vi "Simple TCP - Server.vi"() -> ()   [LabVIEW 2020]
doc: "Demonstrates how to set up a basic TCP connection, send data to the specified port once a connection has been established, and terminate the connection once the data has been sent. This VI is designed to stop if the TCP connection is terminated. The data sent in this example is an array of random numbers."
panel:
  out "error out":errorcluster
  out "x != 0?":bool
  out "state":enum16{"connected", "waiting", "exit"}(ring)
  out "error IO":errorcluster
  in  "Stop":bool
  out "Loop":i32
  # "Overview: Demonstrates the use of the TCP functions to initialize a TCP server that can send data to a client VI.\nInstructions:\n1. Run the VI.\n2. Open Simple TCP - Client.vi and follow the instructions on its front panel. Note that if you wait longer than 30 seconds to do this after running this VI, it will time out.\n3. Click Stop to stop the VI. Note that if you stop the client VI, this VI will stop automatically."
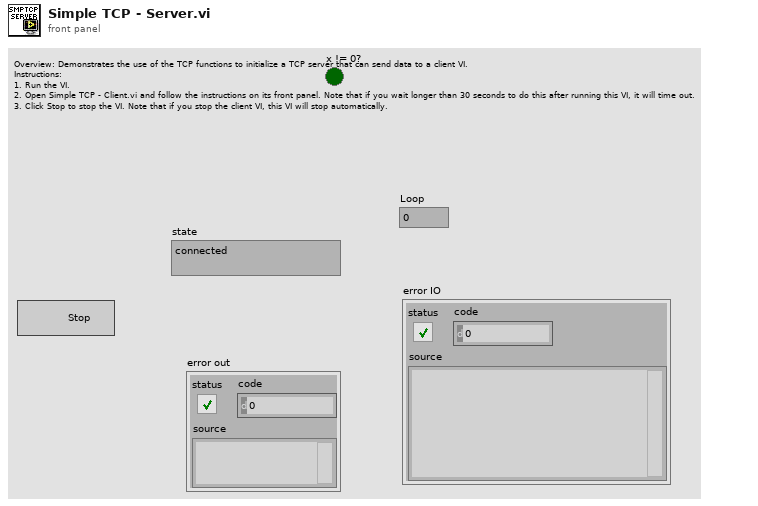
[diagram p1: front panel]
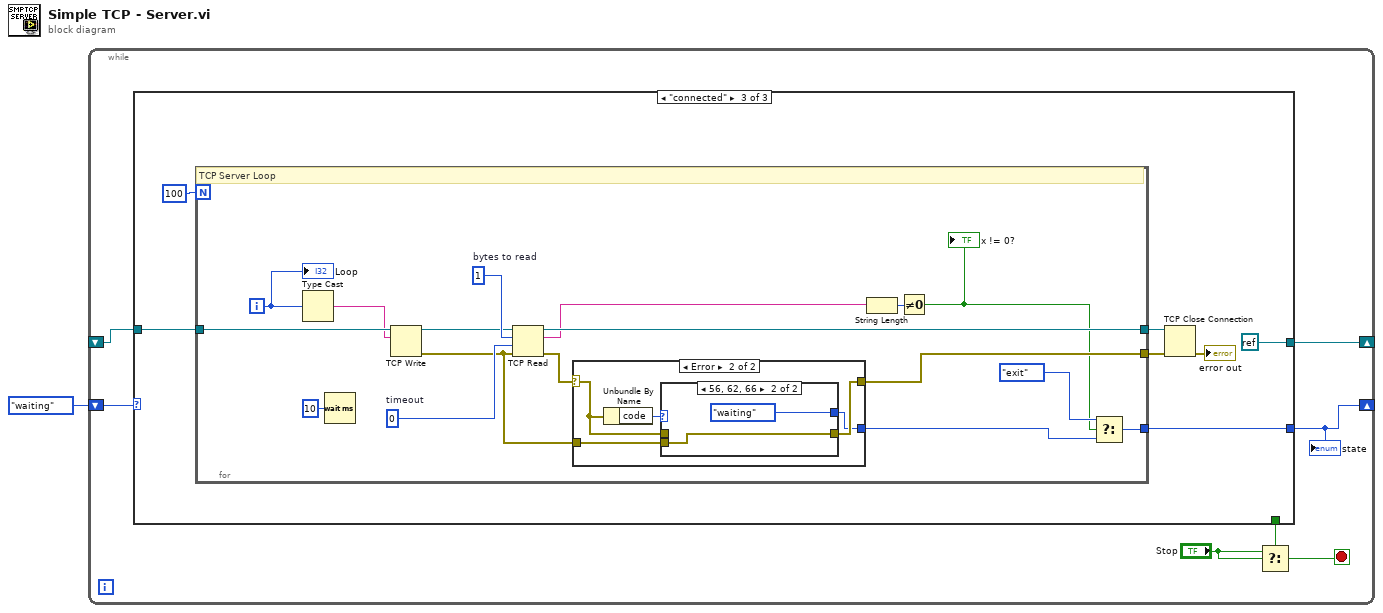
[diagram p0: block diagram]
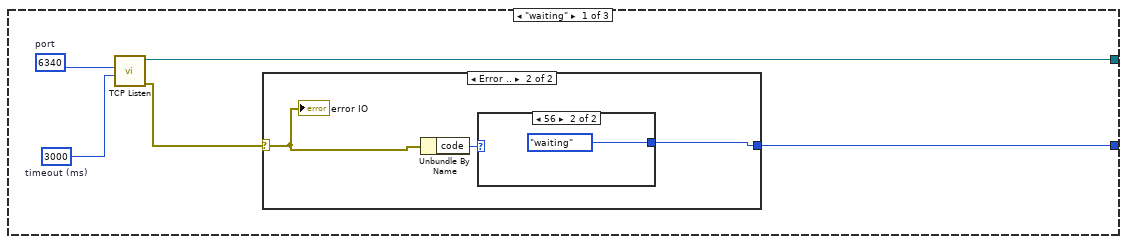
[diagram p2: hidden frame]
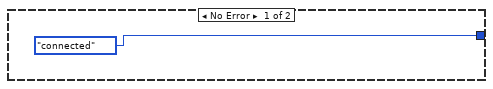
[diagram p3: hidden frame]
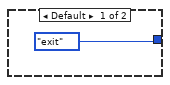
[diagram p4: hidden frame]
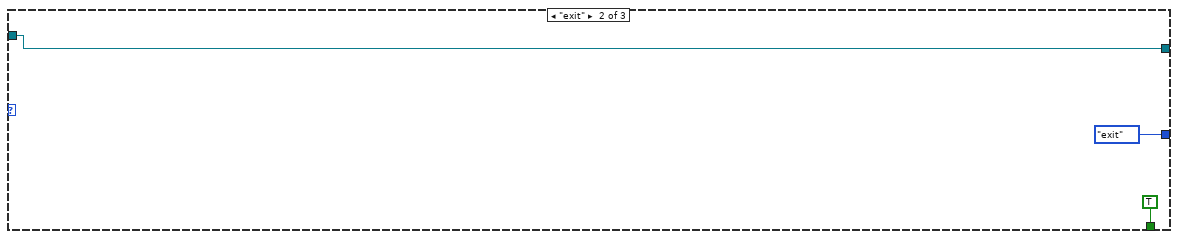
[diagram p5: hidden frame]
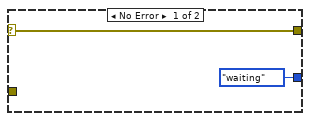
[diagram p6: hidden frame]
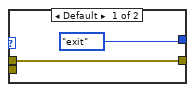
[diagram p7: hidden frame]
diagram:
  n1 = while {
    shift-right: [w4] -> _
    shift-left: enum16{"connected", "waiting", "exit"}."waiting" -> [w8]
    shift-right: [w7] -> _
    shift-left: _ -> [w6]
    stop <- w3 stop-if-true
    n2 = case shown="\"connected\"" w8 {
      tunnel: [w11 w21 refnum<k0> refnum] -> w7
      tunnel: w6 -> [_ w21 w26]
      tunnel: [_ TRUE _] -> w5
      tunnel: [w9 enum16{"connected", "waiting", "exit"}."exit" w24] -> w4
      frame "waiting" {
        w12 = u16 6340  # port
        w13 = 3000  # timeout (ms)
        n3 = call <vilib>:"TCP Listen.vi"("timeout ms (wait forever: -1)"=w13, "port"=w12) -> ("error out"=w10:errorcluster, "connection ID"=w11:refnum<k5>)  [unwired: 5 in, 3 out]
        n4 = case shown="Error .." w10 {
          selector: w10 -> [_ w16]
          tunnel: [enum16{"connected", "waiting", "exit"}."connected" w15] -> w9
          frame No Error {
          }
          frame Error {
            n5 = Unbundle By Name(w16) -> ("code"=w17:i32)
            n6 = case shown="56" w17 {
              tunnel: [enum16{"connected", "waiting", "exit"}."exit" enum16{"connected", "waiting", "exit"}."waiting"] -> w15
              frame Default {
              }
              frame 56 {
              }
            }
            "error IO" <- w16
          }
        }
      }
      frame "exit" {
      }
      frame "connected" {
        n7 = for {
          N: 100 -> [_]
          tunnel: [w36] -> w28
          tunnel: [w41] -> w29
          tunnel: w26 -> [w46]
          tunnel: [w32] -> w24
          i -> [w34]
          w40 = 0  # timeout
          w43 = 1  # bytes to read
          # "TCP Server Loop"
          n8 = Type Cast(x=w34) -> (*(type *) &x=w45:string)  [unwired: 1 out]
          n9 = Wait (ms)(milliseconds to wait=u32 10) -> ()  [unwired: 1 out]
          n10 = TCP Write(connection ID=w46, data in=w45) -> (connection ID out=w42:refnum<k5>, error out=w35:errorcluster)  [unwired: 1 in, 2 out]
          n11 = TCP Read(connection ID=w42, bytes to read=w43, error in (no error)=w35, 9:w40) -> (connection ID out=w41:refnum<k5>, data out=w38:string, error out=w37:errorcluster)  [unwired: 1 out]
          n12 = case shown="Error" w37 {
            selector: w37 -> [w48 w52]
            tunnel: [w48 w50] -> w36
            tunnel: w35 -> [_ w51]
            tunnel: [enum16{"connected", "waiting", "exit"}."waiting" w49] -> w33
            frame No Error {
            }
            frame Error {
              n13 = Unbundle By Name(w52) -> ("code"=w53:i32)
              n14 = case shown="56, 62, 66" w53 {
                tunnel: w52 -> [w55 _]
                tunnel: w51 -> [_ w57]
                tunnel: [w55 w57] -> w50
                tunnel: [enum16{"connected", "waiting", "exit"}."exit" enum16{"connected", "waiting", "exit"}."waiting"] -> w49
                frame Default {
                }
                frame 56, 62, 66 {
                }
              }
            }
          }
          n15 = String Length(string=w38) -> (length=w39:i32)
          n16 = Not Equal To 0?(x=w39) -> (x != 0?=w30:bool)
          "x != 0?" <- w30
          n17 = Select(t=enum16{"connected", "waiting", "exit"}."exit" ("f"), s=w30, f=w33) -> (s? t:f=w32:enum16{"connected", "waiting", "exit"})
          "Loop" <- w34
        }
        n18 = TCP Close Connection(connection ID=w29, error in (no error)=w28) -> (error out=→"error out":errorcluster)  [unwired: 2 out]
      }
    }
    "state" <- w4
    n19 = Select(t="Stop", s="Stop", f=w5) -> (s? t:f=w3:bool)
  }
